vi "safety_range.vi"(1 "ETH Mike Model":T1, 2 "Action (Read)":T2=enum."Read") -> (0 "Safety Range":dbl)   [LabVIEW 2019]
uses:
  ReadOnlyGlobalActions.ctl
  ETHMikeModel.ctl
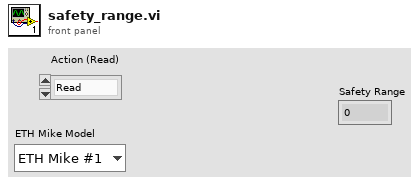
[diagram p1: front panel]
types:
  T1 = typedef "ETHMikeModel.ctl" = enum16{"ETH Mike #1", "ETH Mike #2", "ETH Mike #3", "ETH Mike #4", "ETH MIKE #5"}
  T2 = typedef "ReadOnlyGlobalActions.ctl" = enum16{"Initialize", "Read", "Write"}
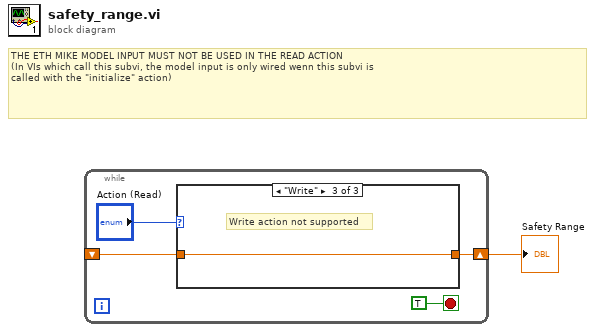
[diagram p0: block diagram]
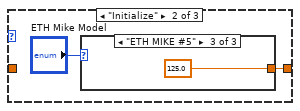
[diagram p3: hidden frame]
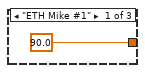
[diagram p4: hidden frame]
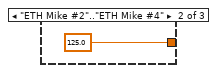
[diagram p5: hidden frame]
diagram:
  # "THE ETH MIKE MODEL INPUT MUST NOT BE USED IN THE READ ACTION\n(In VIs which call this subvi, the model input is only wired wenn this subvi is\ncalled with the \"initialize\" action)"
  n1 = while {
    shift-right: [w4] -> w1
    shift-left: _ -> [w3]
    stop <- TRUE stop-if-true
    n2 = case shown="\"Write\"" "Action (Read)" {
      tunnel: [w6 w7 w12] -> w4
      tunnel: w3 -> [w6 _ w12]
      frame "Read" {
      }
      frame "Initialize" {
        n3 = case shown="\"ETH MIKE #5\"" "ETH Mike Model" {
          tunnel: [90.0 ("I-Part error band") 125.0 ("I-Part error band") 125.0 ("I-Part error band")] -> w7
          frame "ETH Mike #1" {
          }
          frame "ETH Mike #2".."ETH Mike #4" {
          }
          frame "ETH MIKE #5" {
          }
        }
      }
      frame "Write" {
        # "Write action not supported"
      }
    }
  }
  "Safety Range" <- w1
